vi "Agilent DMM Read Event Register.vi"(8 "error in (no error)":errorcluster, 11 "VISA Resource Name":refnum<visa-resource-name>) -> (0 "error out":errorcluster, 2 "Event Register":bool[](array[boolean]), 3 "dup VISA Resource Name":refnum<visa-resource-name>)   [LabVIEW 2011]
doc: "This VI for the HP8753B Network Analyzer reads the status byte and the two event status registers. The two status registers are read out as regular output and will therefore clear anything already in the output queue."
panel:
  # "Operation Complete\n\nNot Used\n\nQuery Error\n\nDevice Error\n\nExecution Error\n\nCommand Error\n\nNot Used\n\nPower On"
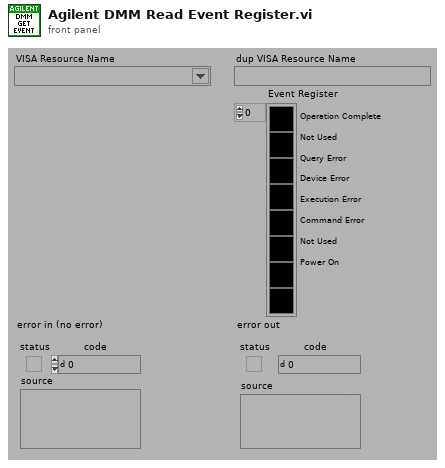
[diagram p1: front panel]
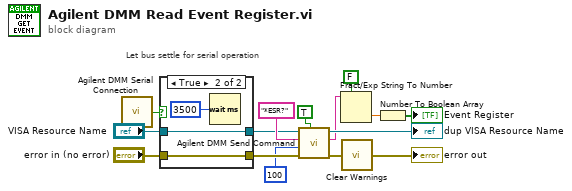
[diagram p0: block diagram]
diagram:
  # "Let bus settle for serial operation"
  n1 = call "Agilent DMM Serial Connection.vi"("VISA Resource Name"="VISA Resource Name") -> ("Serial?"=w10:bool)
  n2 = case shown="True" w10 {
    tunnel: "error in (no error)" -> [w16 w18]
    tunnel: "VISA Resource Name" -> [w17 w19]
    tunnel: [w17 w19] -> w7
    tunnel: [w16 w18] -> w6
    frame False {
    }
    frame True {
      n3 = Wait (ms)(milliseconds to wait=u32 3500) -> ()  [unwired: 1 out]
    }
  }
  n4 = call "Agilent DMM Send Command.vi"("Read? (F)"=TRUE ("use system decimal point (T)"), "error in (no error)"=w6, "Byte Count"=u32 100, "Command"="*ESR?", "VISA Resource Name"=w7) -> ("error out"=w4:errorcluster, "Data Read"=w3:string, "dup VISA Resource Name"=→"dup VISA Resource Name":refnum<visa-resource-name>)  [unwired: 4 out]
  n5 = Fract/Exp String To Number(use system decimal point (T)=FALSE, string=w3) -> (number=w13:dbl)  [unwired: 3 out]
  n6 = call "Clear Warnings.vi"("error in (no error)"=w4) -> ("error out"=→"error out":errorcluster)
  n7 = Number To Boolean Array(number=w13) -> (Boolean array=→"Event Register":bool[])
